vi "Shutdown Metronome.vi"(11 "Actor in":refnum<class "Actor.lvclass">) -> ()   [LabVIEW 2015, in "Actor.lvclass"]
uses:
  Actor.lvclass
  Actor.lvclass/Actor.ctl
  Metronome/API/Metronome Actor API.lvclass
  Utility/Utility.lvlib
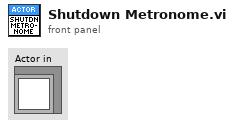
[diagram p1: front panel]
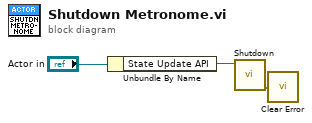
[diagram p0: block diagram]
diagram:
  n1 = Unbundle By Name("Actor in") -> ("State Update API"=w1:refnum<class "Metronome Actor API.lvclass">)
  n2 = call-dynamic "Shutdown.vi"("Actor API in"=w1) -> ("error out"=w2:errorcluster)  [unwired: 10 in]
  n3 = call "Clear Error.vi"("error in (no error)"=w2) -> ()  [unwired: 1 out]
